vi "INIpath.vi"() -> (3 "appended path":path)   [LabVIEW 2017, in "Server.lvlib"]
uses:
  Server.lvlib
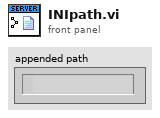
[diagram p1: front panel]
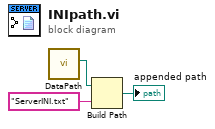
[diagram p0: block diagram]
diagram:
  n1 = call "DataPath.vi"() -> ("DataDirectory"=w3:path)  [unwired: 11 in]
  n2 = Build Path(base path=w3, name or relative path="ServerINI.txt") -> (appended path=→"appended path":path)
